vi "A Position.vi"() -> ()   [LabVIEW 2013]
uses:
  <userlib>/KNR OS 3.0 LabVIEW Toolkit/Type Definition/KNR3 Reference.ctl
  <userlib>/_FPGA Interface Advanced Tools/FPGA Interface Base/FPGA Interface Base.lvclass
  <userlib>/KNR OS 3.0 LabVIEW Toolkit/Type Definition/Resource.ctl
panel:
  out "Circles (Shape Detection 1)":T1(array[cluster]) {"Position"."Y" format="%.2f"; "Position"."X" format="%.2f"}
  out "error out":errorcluster
  out "Number of Matches (Shape Detection 1)":i32
  out "KNR out 4":T2
  in  "Error":errorcluster
  in  "KNR in":T2
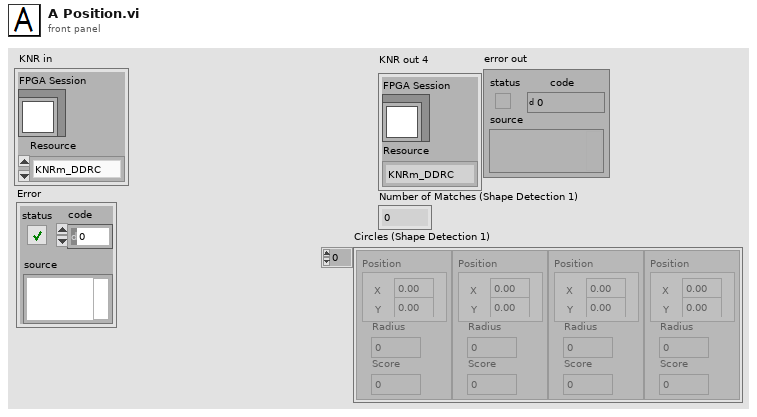
[diagram p1: front panel]
types:
  T1 = cluster{"Position":cluster{"X":sgl, "Y":sgl}, "Radius":dbl, "Score":dbl}[]
  T2 = typedef "KNR3 Reference.ctl" = cluster{"FPGA Session":refnum<class "FPGA Interface Base.lvclass">, "Resource":T3}
  T3 = typedef "Resource.ctl" = enum16{"KNRm_DDRC", "KNRm_DDDD", "KNRm_DDDR", "KNRm_DDDC", "KNR"}
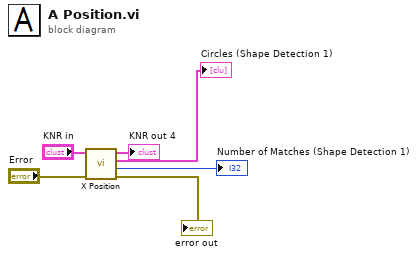
[diagram p0: block diagram]
diagram:
  n1 = call "X Position.vi"("Error"="Error", "KNR in"="KNR in") -> ("error out"=→"error out":errorcluster, "Number of Matches (Shape Detection 1)"=→"Number of Matches (Shape Detection 1)":i32, "Circles (Shape Detection 1)"=→"Circles (Shape Detection 1)":T1, "KNR out 4"=→"KNR out 4":T2)  [unwired: 5 in, 1 out]
